vi "Add channel to Maps for PWM Tags.vi"(7 "engine configuration in":refnum<class "engine configuration.lvclass">, 9 "Tag Name In":string, 10 "Mappings in":T1 {"Line"."Parameters"."Voltage Config"."out terminal configuration (V)" items=["Default"=-1, "RSE"=10083, "Differential"=10106, "Pseudodifferential"=12529]; "Line"."Parameters"."Voltage Config"."in terminal configuration (V)" items=["Default"=-1, "RSE"=10083, "NRSE"=10078, "Differential"=10106, "Pseudodifferential"=12529]; "Line"."Parameters"."Current Config"."shunt resistor location" items=["default"=-1, "Internal"=10200, "External"=10167]; "Line"."Parameters"."Current Config"."input terminal configuration (C)" items=["default"=-1, "RSE"=10083, "NRSE"=10078, "Differential"=10106, "Pseudodifferential"=12529]; "Line"."Parameters"."RTD Config"."resistance configuration" items=["2-Wire"=2, "3-Wire"=3, "4-Wire"=4]; "Line"."Parameters"."RTD Config"."rtd type" items=["Pt3750"=12481, "Pt3851"=10071, "Pt3911"=12482, "Pt3916"=10069, "Pt3920"=10053, "Pt3928"=12483, "Custom"=10137]; "Line"."Parameters"."RTD Config"."current excitation source" items=["Internal"=10200, "External"=10167, "None"=10230]; "Line"."Parameters"."Thermocouple Config"."thermocouple type" items=["J"=10072, "K"=10073, "N"=10077, "R"=10082, "S"=10085, "T"=10086, "B"=10047, "E"=10055]; "Line"."Parameters"."Thermocouple Config"."cjc source" items=["Built-In"=10200, "Constant Value"=10116, "Channel"=10113]; "Line"."Parameters"."Strain Config"."bridge information"."strain configuration" items=["Full Bridge I"=10183, "Full Bridge II"=10184, "Full Bridge III"=10185, "Half Bridge I"=10188, "Half Bridge II"=10189, "Quarter Bridge I"=10271, "Quarter Bridge II"=10272]; "Line"."Parameters"."Strain Config"."bridge information"."voltage excitation source" items=["Internal"=10200, "External"=10167, "None"=10230]}, 11 "Index":i32) -> (2 "Full Tag List":string[](array[string]), 3 "Mappings out":T1 {"Line"."Parameters"."Voltage Config"."out terminal configuration (V)" items=["Default"=-1, "RSE"=10083, "Differential"=10106, "Pseudodifferential"=12529]; "Line"."Parameters"."Voltage Config"."in terminal configuration (V)" items=["Default"=-1, "RSE"=10083, "NRSE"=10078, "Differential"=10106, "Pseudodifferential"=12529]; "Line"."Parameters"."Current Config"."shunt resistor location" items=["default"=-1, "Internal"=10200, "External"=10167]; "Line"."Parameters"."Current Config"."input terminal configuration (C)" items=["default"=-1, "RSE"=10083, "NRSE"=10078, "Differential"=10106, "Pseudodifferential"=12529]; "Line"."Parameters"."RTD Config"."resistance configuration" items=["2-Wire"=2, "3-Wire"=3, "4-Wire"=4]; "Line"."Parameters"."RTD Config"."rtd type" items=["Pt3750"=12481, "Pt3851"=10071, "Pt3911"=12482, "Pt3916"=10069, "Pt3920"=10053, "Pt3928"=12483, "Custom"=10137]; "Line"."Parameters"."RTD Config"."current excitation source" items=["Internal"=10200, "External"=10167, "None"=10230]; "Line"."Parameters"."Thermocouple Config"."thermocouple type" items=["J"=10072, "K"=10073, "N"=10077, "R"=10082, "S"=10085, "T"=10086, "B"=10047, "E"=10055]; "Line"."Parameters"."Thermocouple Config"."cjc source" items=["Built-In"=10200, "Constant Value"=10116, "Channel"=10113]; "Line"."Parameters"."Strain Config"."bridge information"."strain configuration" items=["Full Bridge I"=10183, "Full Bridge II"=10184, "Full Bridge III"=10185, "Half Bridge I"=10188, "Half Bridge II"=10189, "Quarter Bridge I"=10271, "Quarter Bridge II"=10272]; "Line"."Parameters"."Strain Config"."bridge information"."voltage excitation source" items=["Internal"=10200, "External"=10167, "None"=10230]})   [LabVIEW 2015, in "DAQmx Module editor node.lvclass"]
uses:
  DAQmx Module editor node.lvclass
  Mappings.ctl
  module/configuration/Line.ctl
  <vilib>/NI/Tag Bus Module Framework/channel/TBM channel.lvclass
  module/configuration/Measurement Type.ctl
  module/configuration/Parameters.ctl
  Map.ctl
  <vilib>/NI/Module Execution Interface/Engine Configuration/engine configuration.lvclass
  <vilib>/NI/Tag Bus/tag/tag descriptor.lvclass/tag descriptor.ctl
  <vilib>/NI/Tag Bus/tag/tag descriptor.lvclass
  module/configuration/Daqmx Module configuration.lvclass
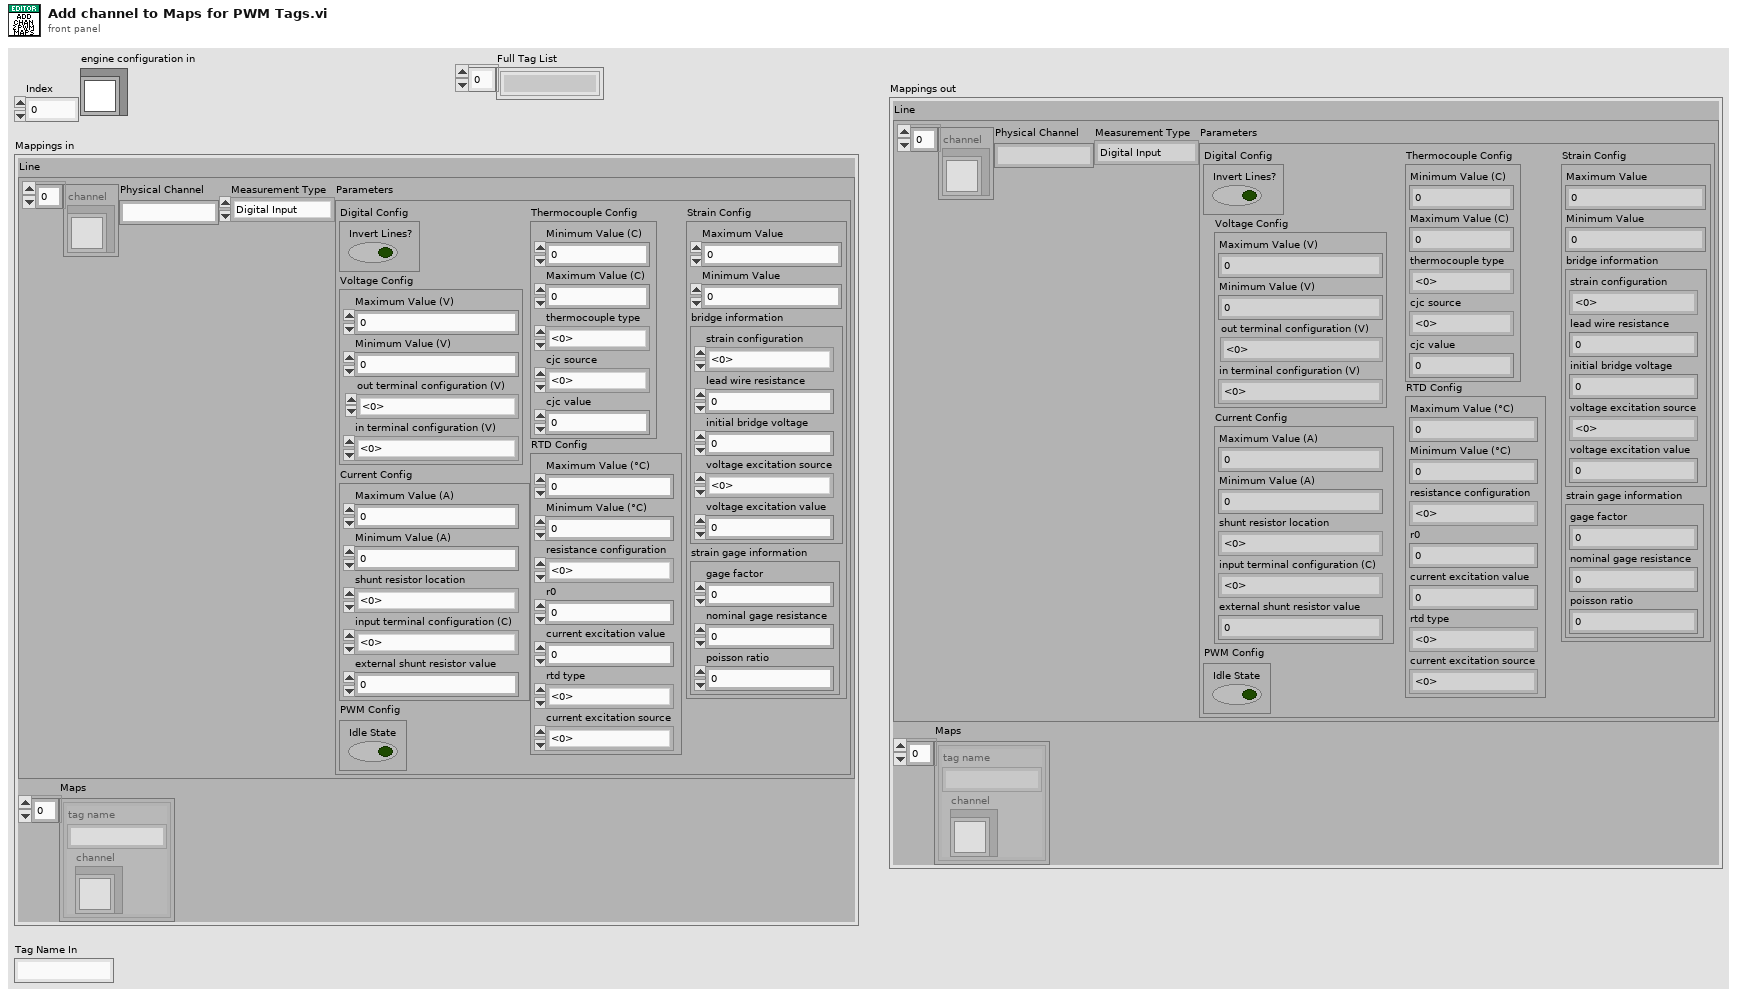
[diagram p1: front panel]
types:
  T1 = typedef "DAQmx Module editor node.lvclass/Mappings.ctl" = cluster{"Line":T2, "Maps":T5[]}
  T2 = typedef "DAQmx Module Configuration.lvclass/Line.ctl" = cluster{"Channel Array":refnum<class "TBM channel.lvclass">[], "Physical Channel":string, "Measurement Type":T3, "Parameters":T4}
  T3 = typedef "DAQmx Module Configuration.lvclass/Measurement Type.ctl" = enum16{"Digital Input", "Digital Output", "Voltage Input", "Voltage Output", "Current Input", "Current Output", "RTD", "Thermocouple", "Strain", "PWM"}
  T4 = typedef "DAQmx Module Configuration.lvclass/Parameters.ctl" = cluster{"Digital Config":cluster{"Invert Lines?":bool}, "Voltage Config":cluster{"Maximum Value (V)":dbl, "Minimum Value (V)":dbl, "in terminal configuration (V)":i32, "out terminal configuration (V)":i32}, "Current Config":cluster{"Maximum Value (A)":dbl, "Minimum Value (A)":dbl, "shunt resistor location":i32, "input terminal configuration (C)":i32, "external shunt resistor value":dbl}, "RTD Config":cluster{"Maximum Value (°C)":dbl, "Minimum Value (°C)":dbl, "resistance configuration":i32, "r0":dbl, "current excitation value":dbl, "rtd type":i32, "current excitation source":i32}, "Thermocouple Config":cluster{"Minimum Value (C)":dbl, "Maximum Value (C)":dbl, "thermocouple type":i32, "cjc source":i32, "cjc value":dbl}, "Strain Config":cluster{"Maximum Value":dbl, "Minimum Value":dbl, "bridge information":cluster{"strain configuration":i32, "lead wire resistance":dbl, "initial bridge voltage":dbl, "voltage excitation source":i32, "voltage excitation value":dbl}, "strain gage information":cluster{"gage factor":dbl, "nominal gage resistance":dbl, "poisson ratio":dbl}}, "PWM Config":cluster{"Idle State":bool}}
  T5 = typedef "DAQmx Module editor node.lvclass/Map.ctl" = cluster{"channel":refnum<class "TBM channel.lvclass">, "tag name":string}
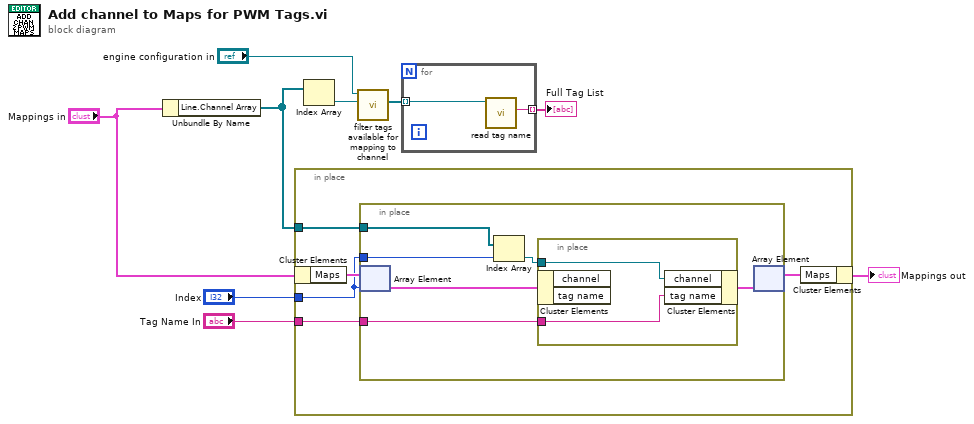
[diagram p0: block diagram]
diagram:
  n1 = Unbundle By Name("Mappings in") -> ("Line.Channel Array"=w4:refnum<class "TBM channel.lvclass">[])
  n2 = in-place {
    in-place-border: "Index" -> [w12]
    in-place-border: "Tag Name In" -> [w11]
    in-place-border: w4 -> [w10]
    n3 = in-place-cluster #1("Mappings in") -> ("Maps"=w14:T5[])
    n4 = in-place {
      in-place-border: w10 -> [w19]
      in-place-border: w11 -> [w18]
      in-place-border: w12 -> [w16]
      n5 = in-place-array #2(w14, w12) -> (w20:T5)
      n6 = Index Array(array=w19, index=w16) -> (element=w17:refnum<class "TBM channel.lvclass">)
      n7 = in-place {
        in-place-border: w18 -> [w22]
        in-place-border: w17 -> [w21]
        n8 = in-place-cluster #3(w20) -> ()  [unwired: 2 out]
        n9 = in-place-cluster #3("channel"=w21, "tag name"=w22) -> (w15:T5)
      }
      n10 = in-place-array #2(w15) -> (w13:T5[])  [unwired: 1 out]
    }
    n11 = in-place-cluster #1("Maps"=w13) -> (→"Mappings out":T1)
  }
  n12 = Index Array(array=w4) -> (element=w2:refnum<class "TBM channel.lvclass">)  [unwired: 1 in]
  n13 = call-dynamic "filter tags available for mapping to channel.vi"("channel to map to"=w2, "engine configuration in"="engine configuration in") -> ("filtered tags"=w6:refnum<class "tag descriptor.lvclass">[])  [unwired: 8 in, 1 out]
  n14 = for {
    tunnel: w6 -> [w24] mode=indexing
    tunnel: [w23] -> w1 mode=indexing
    n15 = call <vilib>:"read tag name.vi"("system tag in"=w24) -> ("name"=w23:string)  [unwired: 8 in, 2 out]
  }
  "Full Tag List" <- w1
